vi "ParsingRangeBitsOfByte.vi"(9 "num bits":u8, 10 "start bit":u8, 11 "value":u64) -> (3 "result":u32)   [LabVIEW 2018, in "Library-DataConvert.lvlib"]
uses:
  Library-DataConvert.lvlib
panel:
  out "불리언 배열":bool[](array[boolean])
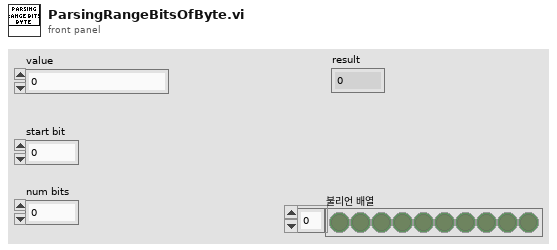
[diagram p1: front panel]
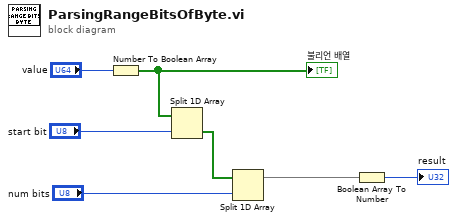
[diagram p0: block diagram]
diagram:
  n1 = Number To Boolean Array(number="value") -> (Boolean array=w6:bool[])
  "불리언 배열" <- w6
  n2 = Split 1D Array(array=w6, index="start bit") -> (second subarray=w4:bool[])  [unwired: 1 out]
  n3 = Split 1D Array(array=w4, index="num bits") -> (first subarray=w2:bool[])  [unwired: 1 out]
  n4 = Boolean Array To Number(Boolean array=w2) -> (number=→"result":u32)
